vi "Periodic Tasks.vi"(8 "error in":errorcluster) -> ()   [LabVIEW 2013]
doc: "This VI runs in parallel to other tasks. It can contain as many user-defined periodic loops as you need. These can carry out PID or other sorts of timed response."
uses:
  <vilib>/Rock Robotics/SystemInterfaces/Utilities/FPGA_UtilitiesLED Source.ctl
  <vilib>/Rock Robotics/SystemInterfaces/Utilities/FPGA_UtilitiesLED State.ctl
  Robot Global Data.vi
  <vilib>/Rock Robotics/WPI/RobotDrive/WPI_RobotDriveGetSetRefNum.vi
  <vilib>/Rock Robotics/WPI/Joystick/WPI_JoystickGetSetRefNum.vi
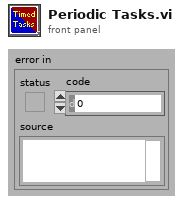
[diagram p1: front panel]
types:
  T1 = typedef "FPGA_UtilitiesLED State.ctl" = enum16{"Off", "On", "Toggle"}
  T2 = typedef "FPGA_UtilitiesLED Source.ctl" = enum16{"User LED", "FPGA LED"}
  T3 = typedef "WPI_DigitalOutputDevRef.ctl" = cluster{"Digital Module":T4, "DIO Channel":T5, "DevStatus":errorcluster}
  T4 = typedef "FPGA_TypedefDigitalModule.ctl" = enum16{"Digital Module 1", "Digital Module 2"}
  T5 = typedef "FPGA_DIOChannel.ctl" = enum8{"DIO 1", "DIO 2", "DIO 3", "DIO 4", "DIO 5", "DIO 6", "DIO 7", "DIO 8", "DIO 9", "DIO 10", "DIO 11", "DIO 12", "DIO 13", "DIO 14", "Invalid"}
  T6 = typedef "WPI_JoystickDevRef.ctl" = cluster{"Device":T7}
  T7 = typedef "WPI_JoystickDeviceEnum.ctl" = enum16{"USB 1", "USB 2", "USB 3", "USB 4", "Kinect 1", "Kinect 2"}
  T8 = typedef "WPI_RobotDriveDevRef.ctl" = cluster{"DevStatus":errorcluster, "Motors[]":T9[], "Square Inputs":bool, "Max Output":dbl, "Isochronous":bool}
  T9 = typedef "WPI_MotorControlDeviceRef.ctl" = cluster{"DeviceStatus":errorcluster, "Type":enum16{"PWM", "CAN"}, "PWM":cluster{"Digital Module":T4, "PWM Channel":T10, "DeadBand":T11}, "CAN":cluster{"Device Number":u8, "Control Mode":T12, "Semaphore":T13, "Max Vout":dbl}, "Invert":bool, "TransformRef":T14, "InvTransformRef":T14}
  T10 = typedef "FPGA_DIOPWMChannel.ctl" = enum8{"PWM 1", "PWM 2", "PWM 3", "PWM 4", "PWM 5", "PWM 6", "PWM 7", "PWM 8", "PWM 9", "PWM 10", "Invalid"}
  T11 = typedef "WPI_PWMDeadband.ctl" = cluster{"Name":string, "maxPositivePwm":i32, "minPositivePwm":i32, "centerPwm":i32, "maxNegativePwm":i32, "minNegativePwm":i32, "angularRange":u16}
  T12 = typedef "WPI_CANJaguar_ControlMode.ctl" = enum8{"Percent VBus", "Current", "Speed", "Position", "Voltage"}
  T13 = typedef "Semaphore RefNum" = refnum<k1>
  T14 = typedef "WPI_PWMTransform_ConPane.ctl" = refnum<vi>
  T15 = cluster{"JoystickDevRef":T6, "RobotDriveDevRef":T8}
  T16 = typedef "WPI_PWMDeviceRef.ctl" = cluster{"DeviceStatus":errorcluster, "Digital Module":T4, "PWM Channel":T10}
  T17 = typedef "WPI_JoystickButtonState.ctl" = cluster{"Button 1":bool, "Button 2":bool, "Button 3":bool, "Button 4":bool, "Button 5":bool, "Button 6":bool, "Button 7":bool, "Button 8":bool, "Button 9":bool, "Button 10":bool, "Button 11":bool, "Button 12":bool}
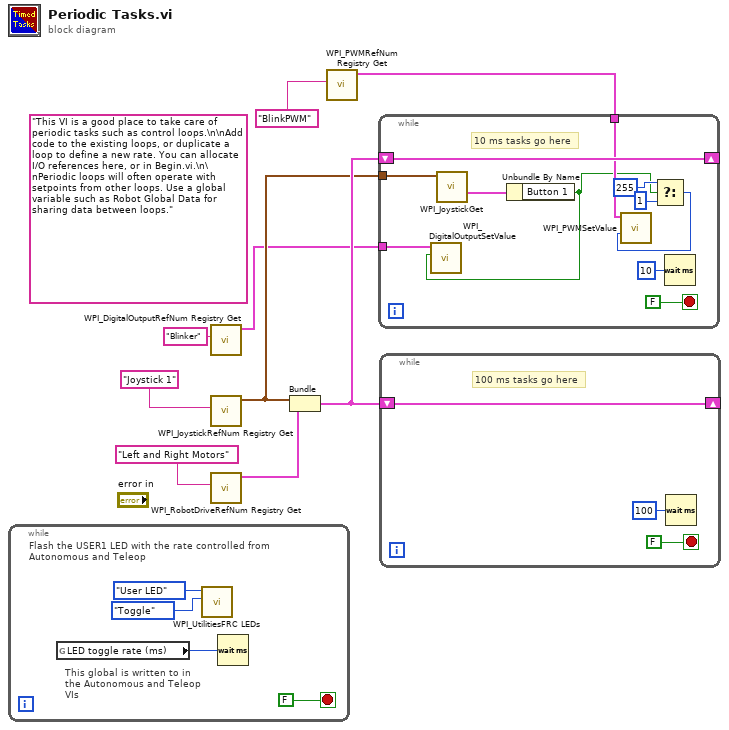
[diagram p0: block diagram]
diagram:
  (unwired) "This VI is a good place to take care of periodic tasks such as control loops.\n\nAdd code to the existing loops, or duplicate a loop to define a new rate. You can allocate I/O references here, or in Begin.vi.\n\nPeriodic loops will often operate with setpoints from other loops. Use a global variable such as Robot Global Data for sharing data between loops."
  n1 = while {
    stop <- FALSE stop-if-true
    # "This global is written to in the Autonomous and Teleop VIs"
    # "Flash the USER1 LED with the rate controlled from Autonomous and Teleop"
    n2 = global read "Robot Global Data.vi" "LED toggle rate (ms)"() -> (w10:u32)
    n3 = call <vilib>:"WPI_UtilitiesFRC LEDs.vi"("State"=FPGA_UtilitiesLED_State."Toggle", "LED Type"=FPGA_UtilitiesLED_Source."User LED") -> ()  [unwired: 1 in, 9 out]
    n4 = Wait (ms)(milliseconds to wait=w10) -> ()  [unwired: 1 out]
  }
  n5 = call <vilib>:"WPI_DigitalOutputRefNum Registry Get.vi"("refnum name"="Blinker") -> ("DigitalOutputDevRef"=w4:T3)  [unwired: 9 in, 1 out]
  n6 = call <vilib>:"WPI_JoystickRefNum Registry Get.vi"("refnum name"="Joystick 1") -> ("JoystickDevRef"=w5:T6)  [unwired: 1 in, 9 out]
  n7 = call <vilib>:"WPI_RobotDriveRefNum Registry Get.vi"("refnum name"="Left and Right Motors") -> ("RobotDriveDevRef"=w7:T8)  [unwired: 1 in, 9 out]
  n8 = Bundle("JoystickDevRef"=w5, "RobotDriveDevRef"=w7) -> (w6:T15)  [unwired: 1 out]
  n9 = call <vilib>:"WPI_PWMRefNum Registry Get.vi"("refnum name"="BlinkPWM") -> ("PWMDeviceRef"=w1:T16)  [unwired: 9 in, 1 out]
  n10 = while {
    shift-right: [w22] -> _
    shift-left: w6 -> [w22]
    tunnel: w5 -> [w20]
    tunnel: w4 -> [w19]
    tunnel: w1 -> [w16]
    stop <- FALSE stop-if-true
    # "10 ms tasks go here"
    n11 = call <vilib>:"WPI_JoystickGet.vi"("JoystickDevRef"=w20) -> ("Buttons"=w21:T17)  [unwired: 4 in, 2 out]
    n12 = Unbundle By Name(w21) -> ("Button 1"=w15:bool)
    n13 = call <vilib>:"WPI_DigitalOutputSetValue.vi"("Value"=w15, "DigitalOutputDevRef"=w19) -> ()  [unwired: 8 in, 2 out]
    n14 = Select(t=u8 255 ("Value"), s=w15, f=u8 1 ("Value")) -> (s? t:f=w14:u8)
    n15 = call <vilib>:"WPI_PWMSetValue.vi"("Value"=w14, "PWMDeviceRef"=w16) -> ()  [unwired: 8 in, 2 out]
    n16 = Wait (ms)(milliseconds to wait=u32 10) -> ()  [unwired: 1 out]
  }
  n17 = while {
    shift-right: [w25] -> _
    shift-left: w6 -> [w25]
    stop <- FALSE stop-if-true
    # "100 ms tasks go here"
    n18 = Wait (ms)(milliseconds to wait=u32 100) -> ()  [unwired: 1 out]
  }
